vi "Initialize.vi"(8 "error in":errorcluster, 11 "Network Master in":refnum<class "Network Master.lvclass">) -> (0 "error out":errorcluster, 3 "Network Master out":refnum<class "Network Master.lvclass">)   [LabVIEW 2021, in "Network Master.lvclass"]
doc: "This provides an interface for the master to open a connection to the slave."
uses:
  Network Master.lvclass
  Network Master.lvclass/Network Master.ctl
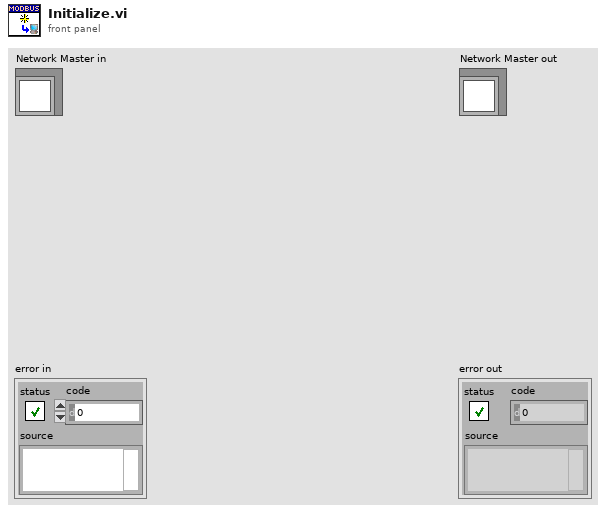
[diagram p1: front panel]
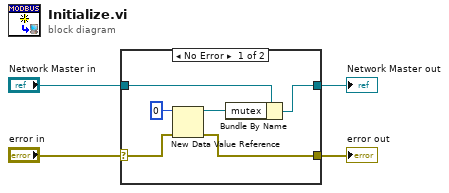
[diagram p0: block diagram]
diagram:
  n1 = case shown="No Error" "error in" {
    selector: "error in" -> [w5 w12]
    tunnel: "Network Master in" -> [w8 w11]
    tunnel: [w7 w11] -> w3
    tunnel: [w6 w12] -> w2
    frame No Error {
      n2 = New Data Value Reference(data value=u8 0, error in=w5) -> (data value reference=w9:refnum<data-value>, error out=w6:errorcluster)
      n3 = Bundle By Name(cluster=w8, "mutex"=w9) -> (w7:refnum<class "Network Master.lvclass">)
    }
    frame Error {
    }
  }
  "error out" <- w2
  "Network Master out" <- w3
